vi "限速.vi"(10 "最大值":dbl=32768.0, 11 "输入":dbl[](array[numeric])) -> (3 "数组":dbl[](array[numeric]))   [LabVIEW 2017]
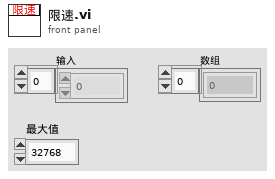
[diagram p1: front panel]
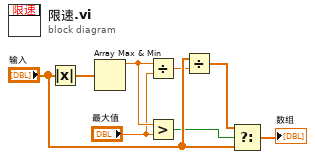
[diagram p0: block diagram]
diagram:
  n1 = Absolute Value(x="输入") -> (abs(x)=w3:dbl[])
  n2 = Array Max & Min(array=w3) -> (max value=w6:dbl)  [unwired: 3 out]
  n3 = Divide(x=w6, y="最大值") -> (x/y=w7:dbl)
  n4 = Greater?(x=w6, y="最大值") -> (0:w5:bool)
  n5 = Divide(x="输入", y=w7) -> (x/y=w4:dbl[])
  n6 = Select(t=w4, s=w5, f="输入") -> (s? t:f=→"数组":dbl[])
